vi "Relink Parallel Subroutine.vi"(4 "Path Builder":refnum<class "IPath Builder.lvclass">, 6 "Persistence in":refnum<class "IPersist.lvclass">, 7 "Linked List ID":string, 8 "error in (no error)":errorcluster, 9 "Return":string, 10 "Paths":path[](array[path]), 11 "Linked List Ref":refnum<data-value>) -> (0 "error out":errorcluster, 1 "Return out":string, 3 "Linked List Ref out":refnum<data-value>)   [LabVIEW 2017]
uses:
  linked-list/Source/Linked List/ILinkedList/ILinked List.lvclass
  persistence/source/IPersist/IPersist.lvclass
  Path Builder/IPath Builder/IPath Builder.lvclass
  ITestExecutive/ITest Executive.lvclass
  TestExecutive/Test Executive.lvclass
  C:/Users/jonmc/Documents/Git/Test Executive/Source/Test Executive/ITestExecutive/ITest Executive.lvclass
  807f29ff-2c0d-4845-96e3-26f7bacf8274.vi
  0686657e-ce3c-4cb1-8915-926bffe558a0.vi
  ca3b3864-f623-498d-896c-89439c00b138.vi
  ebd35830-aab3-4a8c-9439-be88075cf000.vi
  07fadd7c-f439-428d-8b7d-a5d48cbb0b9a.vi
  60a4713c-9991-498e-b8cc-026215c46d89.vi
  350e5f9f-4912-4a60-9d4e-228846dd99f0.vi
  8f5accf5-3a0b-49c7-8256-3e71f9fad646.vi
  9afac329-2102-4699-842b-ef5eac783a5a.vi
  <vilib>/Utility/error.llb/Error Cluster From Error Code.vi
  linked-list/Source/Linked List/Linked List Ref/Linked List Ref.lvclass
  TestExecutive Ref/TestExecutive Ref.lvclass
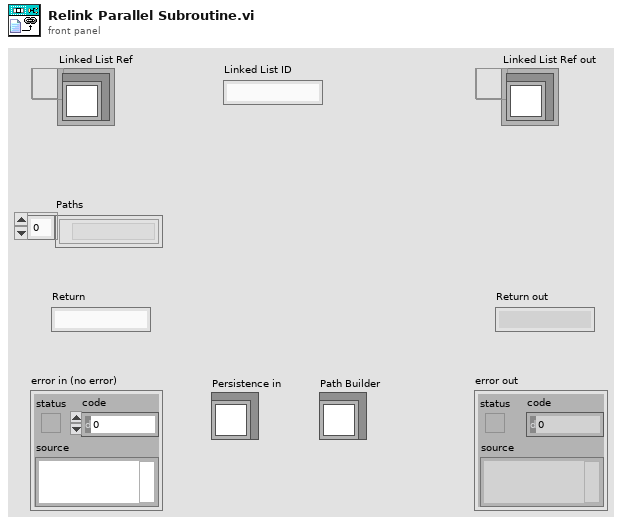
[diagram p1: front panel]
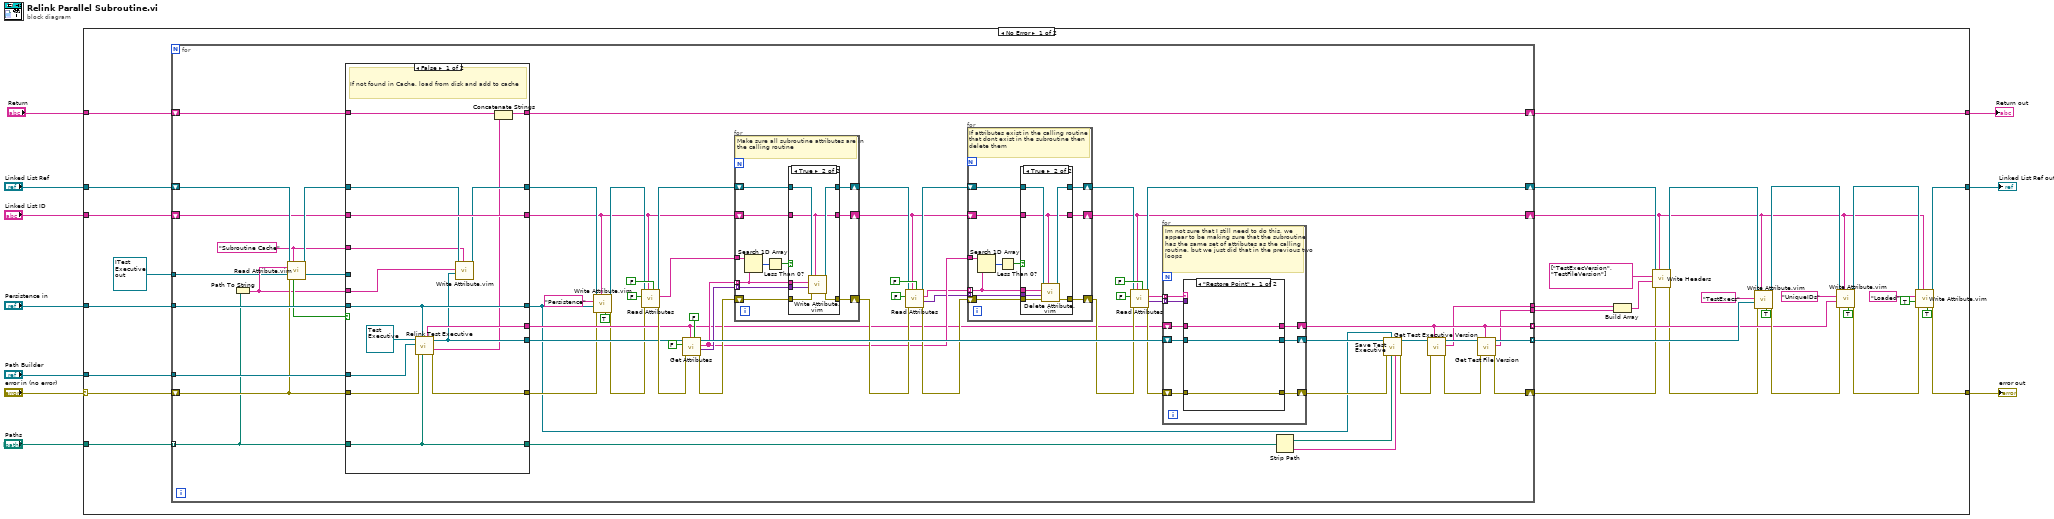
[diagram p0: block diagram]
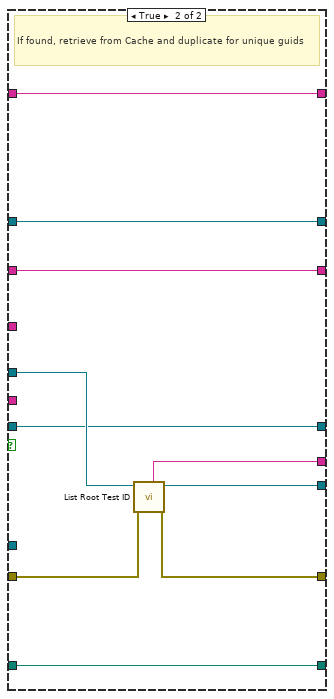
[diagram p2: hidden frame]
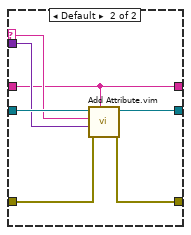
[diagram p5: hidden frame]
diagram:
  n1 = case shown="No Error" "error in (no error)" {
    selector: "error in (no error)" -> [w40 w198]
    tunnel: "Persistence in" -> [w43 _]
    tunnel: "Paths" -> [w39 _]
    tunnel: "Path Builder" -> [w42 _]
    tunnel: "Linked List Ref" -> [w41 w199]
    tunnel: "Linked List ID" -> [w38 _]
    tunnel: [w25 w199] -> w4
    tunnel: [w24 w198] -> w5
    tunnel: "Return" -> [w21 w197]
    tunnel: [w20 w197] -> w1
    frame No Error {
      n2 = for {
        tunnel: w43 -> [w110]
        tunnel: w42 -> [w109]
        tunnel: w39 -> [w79] mode=indexing
        tunnel: [w51] -> w22 mode=indexing
        shift-right: [w69] -> w17
        shift-left: w41 -> [w81]
        shift-right: [w47] -> w12
        shift-left: w40 -> [w80]
        shift-right: [w68] -> w15
        shift-left: w38 -> [w76]
        tunnel: refnum<data-value> refnum ("Test Executive Ref out") -> [w73]
        tunnel: [w52] -> w23 mode=indexing
        shift-right: [w58] -> w20
        shift-left: w21 -> [w59]
        tunnel: [w45] -> w14
        tunnel: [w44] -> w13
        w74 = "Subroutine Cache" ("Name")
        n3 = Path To String(path=w79) -> (string=w75:string)
        n4 = call "Read Attribute.vim"("Linked List Ref"=w81, "Linked List ID"=w74, "Attribute Name"=w75, "Type"=w73, "error in (no error)"=w80) -> ("Linked List Ref out"=w77:refnum<data-value>, "Attribute"=w72:refnum<data-value>, "Found?"=w78:bool)  [unwired: 5 in, 3 out]
        n5 = case shown="False" w78 {
          tunnel: [w115 w133] -> w64
          tunnel: w110 -> [w121 w129]
          tunnel: w109 -> [w118 _]
          tunnel: [w114 w131] -> w71
          tunnel: [w120 w130] -> w70
          tunnel: w80 -> [w117 w134]
          tunnel: w79 -> [w116 w128]
          tunnel: [w124 w136] -> w62
          tunnel: w77 -> [w125 w136]
          tunnel: [w126 w135] -> w61
          tunnel: w76 -> [w126 w135]
          tunnel: w75 -> [w122 _]
          tunnel: w74 -> [w123 _]
          tunnel: w72 -> [_ w132]
          tunnel: [w121 w129] -> w46
          tunnel: [w116 w128] -> w60
          tunnel: w59 -> [w113 w127]
          tunnel: [w111 w127] -> w58
          frame False {
            # "If not found in Cache, load from disk and add to cache"
            n6 = call "Relink Test Executive.vi"("File"=w116, "Persistence in"=w121, "error in (no error)"=w117, "Path Builder"=w118, "Test Executive"=refnum<class "Test Executive.lvclass"> refnum ("Test Executive.lvlib:Test Executive.lvclass")) -> ("error out"=w115:errorcluster, "Return"=w112:string, "Test Executive Ref out"=w114:refnum<data-value>, "Root ID"=w120:string)  [unwired: 3 in]
            n7 = call "Write Attribute.vim"("Linked List ID"=w123, "Attribute"=w114, "Attribute Name"=w122, "Linked List Ref"=w125) -> ("Linked List Ref out"=w124:refnum<data-value>)  [unwired: 4 in, 3 out]
            n8 = Concatenate Strings(w113, w112) -> (w111:string)
          }
          frame True {
            # "If found, retrieve from Cache and duplicate for unique guids"
            n9 = call "List Root Test ID.vi"("error in (no error)"=w134, "Test Executive Ref"=w132) -> ("error out"=w133:errorcluster, "Test Executive Ref out"=w131:refnum<data-value>, "Root ID"=w130:string)  [unwired: 5 in, 2 out]
          }
        }
        n10 = call "Write Attribute.vim"("Private?"=TRUE, "Linked List ID"=w61, "error in (no error)"=w64, "Attribute"=w46, "Attribute Name"="Persistence", "Linked List Ref"=w62) -> ("error out"=w65:errorcluster, "Linked List Ref out"=w63:refnum<data-value>)  [unwired: 2 in, 2 out]
        n11 = call "Read Attributes.vi"("Flatten Pointer?"=FALSE, "Linked List ID"=w61, "error in (no error)"=w65, "Include Private?"=FALSE, "Linked List Ref"=w63) -> ("error out"=w103:errorcluster, "Attribute Names out"=w102:string[], "Linked List Ref out"=w100:refnum<data-value>)  [unwired: 1 in, 3 out]
        n12 = call "Get Attributes.vi"("Flatten Pointer?"=FALSE, "Test ID"=w70, "error in (no error)"=w103, "Include Private?"=FALSE, "Test Executive Ref"=w71) -> ("error out"=w99:errorcluster, "Attributes"=w101:variant[], "Attribute Names out"=w91:string[], "Test Executive Ref out"=w106:refnum<data-value>)  [unwired: 1 in, 2 out]
        n13 = for {
          tunnel: w91 -> [w160] mode=indexing
          tunnel: w101 -> [w159] mode=indexing
          shift-right: [w165] -> w95
          shift-left: w100 -> [w166]
          tunnel: w102 -> [w167]
          shift-right: [w163] -> w96
          shift-left: w99 -> [w164]
          shift-right: [w158] -> w93
          shift-left: w61 -> [w162]
          # "Make sure all subroutine attributes are in the calling routine"
          n14 = Search 1D Array(1D array=w167, element=w160) -> (index of element=w168:i32)  [unwired: 1 in]
          n15 = Less Than 0?(x=w168) -> (x < 0?=w161:bool)
          n16 = case shown="True" w161 {
            tunnel: w166 -> [w171 w178]
            tunnel: [w171 w177] -> w165
            tunnel: w164 -> [w170 w176]
            tunnel: [w170 w175] -> w163
            tunnel: w162 -> [w169 w172]
            tunnel: w160 -> [_ w174]
            tunnel: w159 -> [_ w173]
            tunnel: [w169 w172] -> w158
            frame False {
            }
            frame True {
              n17 = call "Write Attribute.vim"("Linked List ID"=w172, "error in (no error)"=w176, "Attribute"=w173, "Attribute Name"=w174, "Linked List Ref"=w178) -> ("error out"=w175:errorcluster, "Linked List Ref out"=w177:refnum<data-value>)  [unwired: 3 in, 2 out]
            }
          }
        }
        n18 = call "Read Attributes.vi"("Flatten Pointer?"=FALSE, "Linked List ID"=w93, "error in (no error)"=w96, "Include Private?"=FALSE, "Linked List Ref"=w95) -> ("error out"=w92:errorcluster, "Attributes"=w89:variant[], "Attribute Names out"=w90:string[], "Linked List Ref out"=w94:refnum<data-value>)  [unwired: 1 in, 2 out]
        n19 = for {
          tunnel: w90 -> [w139] mode=indexing
          tunnel: w89 -> [w138] mode=indexing
          shift-right: [w144] -> w86
          shift-left: w94 -> [w145]
          tunnel: w91 -> [w146]
          shift-right: [w142] -> w85
          shift-left: w92 -> [w143]
          shift-right: [w137] -> w68
          shift-left: w93 -> [w141]
          # "If attributes exist in the calling routine that dont exist in the subroutine then delete them"
          n20 = Search 1D Array(1D array=w146, element=w139) -> (index of element=w147:i32)  [unwired: 1 in]
          n21 = Less Than 0?(x=w147) -> (x < 0?=w140:bool)
          n22 = case shown="True" w140 {
            tunnel: w145 -> [w150 w157]
            tunnel: [w150 w156] -> w144
            tunnel: w143 -> [w149 w154]
            tunnel: [w149 w153] -> w142
            tunnel: w141 -> [w148 w155]
            tunnel: w139 -> [_ w152]
            tunnel: w138 -> [_ w151]
            tunnel: [w148 w155] -> w137
            frame False {
            }
            frame True {
              n23 = call "Delete Attribute.vim"("Linked List ID"=w155, "error in (no error)"=w154, "Type"=w151, "Attribute Name"=w152, "Linked List Ref"=w157) -> ("error out"=w153:errorcluster, "Linked List Ref out"=w156:refnum<data-value>)  [unwired: 4 in, 1 out]
            }
          }
        }
        n24 = call "Read Attributes.vi"("Flatten Pointer?"=FALSE, "Linked List ID"=w68, "error in (no error)"=w85, "Include Private?"=FALSE, "Linked List Ref"=w86) -> ("error out"=w84:errorcluster, "Attributes"=w83:variant[], "Attribute Names out"=w82:string[], "Linked List Ref out"=w69:refnum<data-value>)  [unwired: 1 in, 2 out]
        n25 = for {
          shift-right: [w183] -> w48
          shift-left: w84 -> [w184]
          tunnel: w82 -> [w182] mode=indexing
          tunnel: w83 -> [w181] mode=indexing
          shift-right: [w180] -> w51
          shift-left: w70 -> [w185]
          shift-right: [w179] -> w53
          shift-left: w106 -> [w186]
          # "Im not sure that I still need to do this, we appear to be making sure that the subroutine has the same set of attributes as the calling routine, but we just did that in the previous two loops"
          n26 = case shown="\"Restore Point\"" w182 {
            selector: w182 -> [_ w193]
            tunnel: w186 -> [w187 w196]
            tunnel: w185 -> [w188 w191]
            tunnel: w184 -> [w189 w195]
            tunnel: [w189 w194] -> w183
            tunnel: w181 -> [_ w192]
            tunnel: [w188 w191] -> w180
            tunnel: [w187 w190] -> w179
            frame "Restore Point" {
            }
            frame Default {
              n27 = call "Add Attribute.vim"("ID"=w191, "error in (no error)"=w195, "Attribute"=w192, "Attribute Name"=w193, "Test Executive Ref"=w196) -> ("error out"=w194:errorcluster, "Test Executive Ref out"=w190:refnum<data-value>)  [unwired: 3 in, 2 out]
            }
          }
        }
        n28 = Strip Path(path=w60) -> (stripped path=w50:path, name=w49:string)
        n29 = call "Save Test Executive.vi"("File Name"=w49, "Folder"=w50, "Persistence in"=w46, "error in (no error)"=w48, "Test Executive Ref"=w53) -> ("error out"=w55:errorcluster, "Test Executive Ref out"=w57:refnum<data-value>)  [unwired: 5 in]
        n30 = call "Get Test Executive Version.vi"("Unique ID"=w51, "error in (no error)"=w55, "Test Executive Ref"=w57) -> ("error out"=w54:errorcluster, "Test Executive Version"=w45:string, "Test Executive Ref out"=w56:refnum<data-value>)  [unwired: 5 in, 1 out]
        n31 = call "Get Test File Version.vi"("Unique ID"=w51, "error in (no error)"=w54, "Test Executive Ref"=w56) -> ("error out"=w47:errorcluster, "Test File Version"=w44:string, "Test Executive Ref out"=w52:refnum<data-value>)  [unwired: 5 in, 1 out]
      }
      n32 = Build Array(w14, w13) -> (w18:string[])
      n33 = call "Write Headers.vi"("Linked List ID"=w15, "error in (no error)"=w12, "Header Values"=w18, "Header Names"=string[] ["TestExecVersion", "TestFileVersion"], "Linked List Ref"=w17) -> ("error out"=w11:errorcluster, "Linked List Ref out"=w16:refnum<data-value>)  [unwired: 5 in]
      n34 = call "Write Attribute.vim"("Private?"=TRUE, "Linked List ID"=w15, "error in (no error)"=w11, "Attribute"=w23, "Attribute Name"="TestExecs", "Linked List Ref"=w16) -> ("error out"=w33:errorcluster, "Linked List Ref out"=w27:refnum<data-value>)  [unwired: 2 in, 2 out]
      n35 = call "Write Attribute.vim"("Private?"=TRUE, "Linked List ID"=w15, "error in (no error)"=w33, "Attribute"=w22, "Attribute Name"="UniqueIDs", "Linked List Ref"=w27) -> ("error out"=w29:errorcluster, "Linked List Ref out"=w26:refnum<data-value>)  [unwired: 2 in, 2 out]
      n36 = call "Write Attribute.vim"("Private?"=TRUE, "Linked List ID"=w15, "error in (no error)"=w29, "Attribute"=TRUE, "Attribute Name"="Loaded", "Linked List Ref"=w26) -> ("error out"=w24:errorcluster, "Linked List Ref out"=w25:refnum<data-value>)  [unwired: 2 in, 2 out]
    }
    frame Error {
    }
  }
  "error out" <- w5
  "Linked List Ref out" <- w4
  "Return out" <- w1
